vi "Get Min_Max_Limits.vi"(6 "Mode":T1=enum."Basic", 7 "[x]":T2, 8 "error in (no error)":errorcluster, 11 "Serial Port in":refnum<visa-resource-name>) -> (0 "error out":errorcluster, 2 "Limits":dbl[](array[numeric]), 3 "Serial Port out":refnum<visa-resource-name>)   [LabVIEW 2020, in "Chemyx_Syringe_Pump_driver.lvlib"]
doc: "Returns the minimum and maximum of volumes and rates of the current pump."
uses:
  Chemyx_Syringe_Pump_driver.lvlib
  _private/Control/Control Mode.ctl
  _private/Control/Programmable Mode.ctl
panel:
  # "Returns the minimum and maximum of volumes and rates of the current pump."
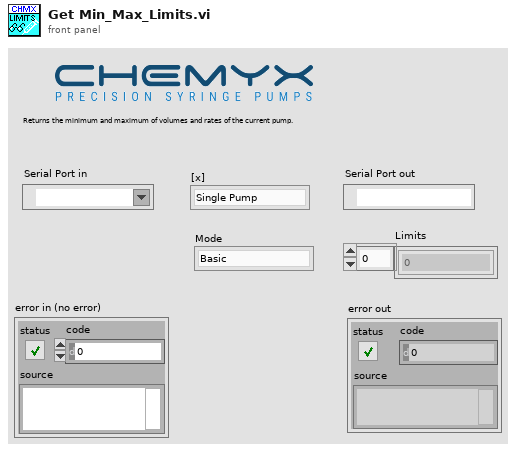
[diagram p1: front panel]
types:
  T1 = typedef "Chemyx_Syringe_Pump_driver.lvlib/Programmable Mode.ctl" = enum16{"Blank", "Basic", "Programmable"}
  T2 = typedef "Chemyx_Syringe_Pump_driver.lvlib/Control Mode.ctl" = enum16{"Single Pump", "Pump Channel 1", "Pump Channel 2", "Cycle Mode"}
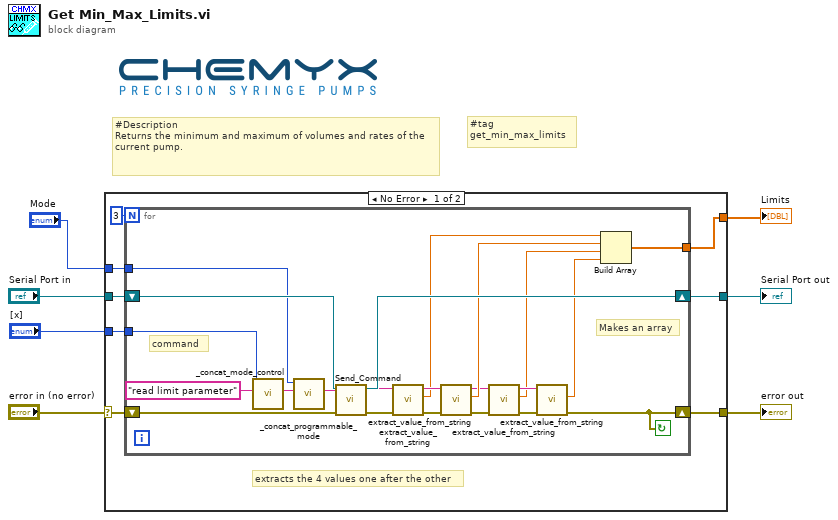
[diagram p0: block diagram]
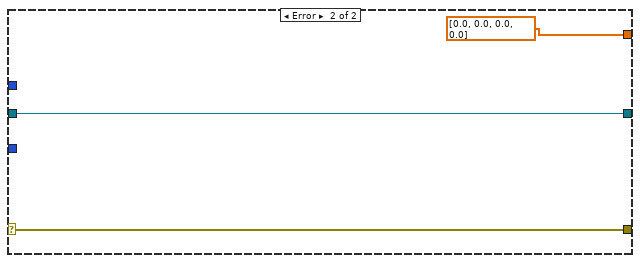
[diagram p2: hidden frame]
diagram:
  # "#tag\nget_min_max_limits"
  # "#Description\nReturns the minimum and maximum of volumes and rates of the current pump."
  n1 = case shown="No Error" "error in (no error)" {
    selector: "error in (no error)" -> [w14 w40]
    tunnel: "Serial Port in" -> [w15 w39]
    tunnel: [w11 w40] -> w5
    tunnel: [w13 w39] -> w4
    tunnel: [w12 dbl[] [0.0, 0.0, 0.0, 0.0]] -> w3
    tunnel: "[x]" -> [w10 _]
    tunnel: "Mode" -> [w9 _]
    frame No Error {
      # "extracts the 4 values one after the other"
      n2 = for {
        N: 3 -> [_]
        tunnel: [w23] -> w12
        tunnel: w10 -> [w20]
        tunnel: w9 -> [w19]
        shift-right: [w35] -> w13
        shift-left: w15 -> [w37]
        shift-right: [w16] -> w11
        shift-left: w14 -> [w36]
        stop <- w16 continue-if-true
        # "Makes an array"
        # "command"
        n3 = call "_concat_mode_control.vi"("write buffer"="read limit parameter", "[x]"=w20) -> ("write buffer out"=w18:string)  [unwired: 9 in]
        n4 = call "_concat_programmable_mode.vi"("write buffer"=w18, "Programmable Mode"=w19) -> ("write buffer out"=w17:string)  [unwired: 9 in]
        n5 = call "Send_Command.vi"("error in (no error)"=w36, "write buffer"=w17, "Serial Port in"=w37) -> ("error out"=w22:errorcluster, "Read buffer"=w34:string, "VISA Refnum out"=w35:refnum<visa-resource-name>)  [unwired: 6 in]
        n6 = call "extract_value_from_string.vi"("error in (no error)"=w22, "Input string"=w34) -> ("error out"=w33:errorcluster, "Value"=w28:dbl, "Rest of string"=w32:string)  [unwired: 7 in]
        n7 = call "extract_value_from_string.vi"("error in (no error)"=w33, "Input string"=w32) -> ("error out"=w31:errorcluster, "Value"=w27:dbl, "Rest of string"=w26:string)  [unwired: 7 in]
        n8 = call "extract_value_from_string.vi"("error in (no error)"=w31, "Input string"=w26) -> ("error out"=w30:errorcluster, "Value"=w25:dbl, "Rest of string"=w29:string)  [unwired: 7 in]
        n9 = call "extract_value_from_string.vi"("error in (no error)"=w30, "Input string"=w29) -> ("error out"=w16:errorcluster, "Value"=w24:dbl)  [unwired: 7 in, 1 out]
        n10 = Build Array(w28, w27, w25, w24) -> (w23:dbl[])
      }
    }
    frame Error {
    }
  }
  "error out" <- w5
  "Serial Port out" <- w4
  "Limits" <- w3
